vi "Write Red.vi"(8 "error in (no error)":errorcluster, 10 "Red":bool, 11 "Laser Enable CMD in":refnum<class "Laser Enable CMD.lvclass">) -> (0 "error out":errorcluster, 3 "Laser Enable CMD out":refnum<class "Laser Enable CMD.lvclass">)   [LabVIEW 2014, in "eCRDS Library.lvlib" / "Laser Enable CMD.lvclass"]
uses:
  Laser Enable CMD.lvclass
  Laser Enable CMD.lvclass/Laser Enable CMD.ctl
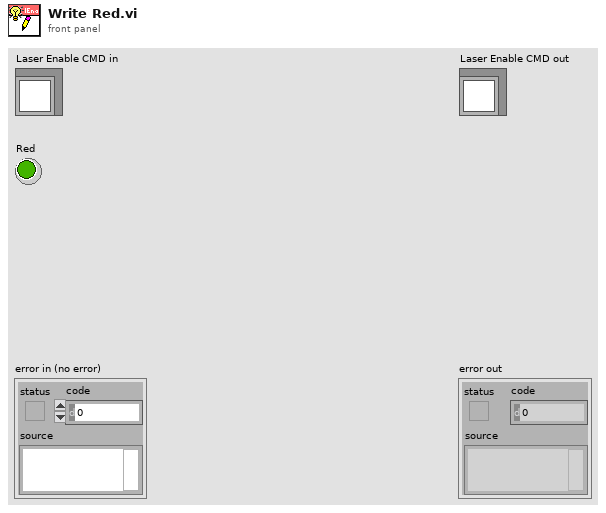
[diagram p1: front panel]
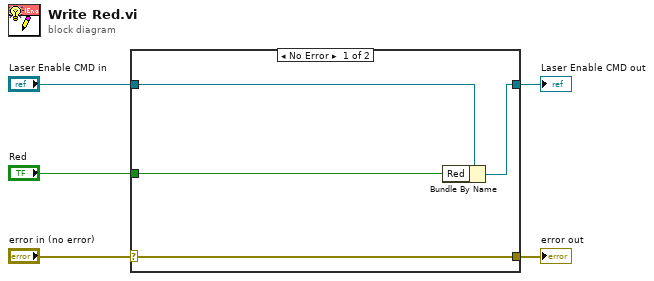
[diagram p0: block diagram]
diagram:
  n1 = case shown="No Error" "error in (no error)" {
    selector: "error in (no error)" -> [w9 w10]
    tunnel: [w9 w10] -> w4
    tunnel: [w7 w11] -> w2
    tunnel: "Laser Enable CMD in" -> [w8 w11]
    tunnel: "Red" -> [w6 _]
    frame No Error {
      n2 = Bundle By Name(cluster=w8, "Red"=w6) -> (w7:refnum<class "Laser Enable CMD.lvclass">)
    }
    frame Error {
    }
  }
  "error out" <- w4
  "Laser Enable CMD out" <- w2
